vi "Read Optional Plane Lines.vi"(9 "XYGraph in":refnum<class "XYGraph.lvclass">) -> (3 "XYGraph out":refnum<class "XYGraph.lvclass">, 4 "Optional Plane Lines":bool)   [LabVIEW 2014, in "XYGraph.lvclass"]
uses:
  XYGraph.lvclass
  XYGraph.lvclass/XYGraph.ctl
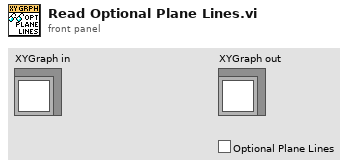
[diagram p1: front panel]
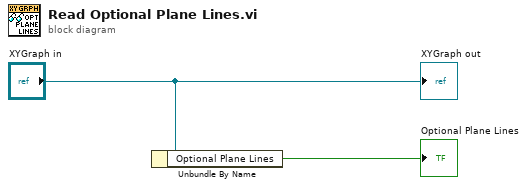
[diagram p0: block diagram]
diagram:
  n1 = Unbundle By Name("XYGraph in") -> ("Optional Plane Lines"=→"Optional Plane Lines":bool)
  "XYGraph out" <- "XYGraph in"
